vi "GT_CloseExtMdl.vi"(1 "rtn_In":cluster{"rtn":i16, "Func":string}) -> (0 "rtn_Out":cluster{"rtn":i16, "Func":string})   [LabVIEW 2014]
uses:
  data/data/ExtMdl.dll
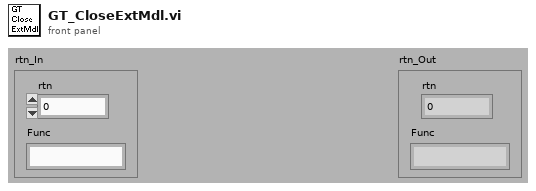
[diagram p1: front panel]
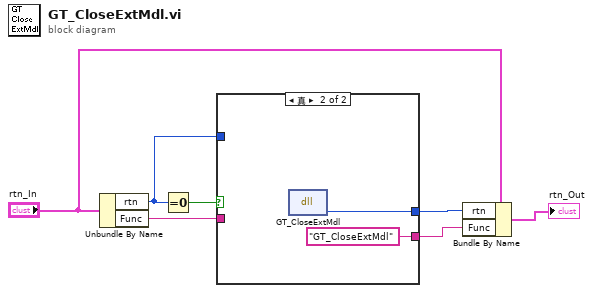
[diagram p0: block diagram]
diagram:
  n1 = Unbundle By Name("rtn_In") -> ("rtn"=w2:i16, "Func"=w1:string)
  n2 = Equal To 0?(x=w2) -> (x = 0?=w7:bool)
  n3 = case shown="真" w7 {
    tunnel: [w9 w11] -> w5
    tunnel: [w8 "GT_CloseExtMdl" ("Func")] -> w3
    tunnel: w2 -> [w9 _]
    tunnel: w1 -> [w8 _]
    frame False {
    }
    frame True {
      n4 = dll-call lib="PTH2Iabs DNewGTS AC-800LWin7版源程序-20170926datadata\nExtMdl.dll" fn="GT_CloseExtMdl"() -> ("rtn"=w11:i32)  [unwired: 3 in, 2 out]
    }
  }
  n5 = Bundle By Name(cluster="rtn_In", "rtn"=w5, "Func"=w3) -> (→"rtn_Out":cluster{"rtn":i16, "Func":string})
